vi "Trabalho.vi"() -> ()   [LabVIEW 2009]
uses:
  <vilib>/NXT/Block Support/NXT_InputPort.ctl
  <vilib>/NXT/Block Support/NXT_ButtonSelector.ctl
  <vilib>/NXT/Subs/MotorOutput.ctl
  <vilib>/NXT/Dual Mode Library/Waits/Wait_Num.vi
  <vilib>/NXT/Dual Mode Library/Display/drawText.vi
  <vilib>/NXT/Dual Mode Library/Sensors/Light_On.vi
  <vilib>/NXT/Dual Mode Library/Sensors/Sound_dB.vi
  <vilib>/NXT/Dual Mode Library/Sensors/Sonar_cm.vi
  <vilib>/NXT/Dual Mode Library/Sensors/readNXTButton.vi
  <vilib>/NXT/Dual Mode Library/Sensors/Touch_Pressed.vi
  <vilib>/NXT/Subs/NXT_SteeringOutputPort.ctl
panel:
  out "Verificacao":bool[](array[boolean])
  out "Cor Inicial":i16
  out "Toque\nPressionado":bool
  out "Visor":string
  out "Ruído":i16(slide) scale=0.0..100.0
  out "Luminosidade":i16
  out "Distância":i16
  out "Botao\nPressionado":bool
  # "O Mindstorms irá ficar no seguinte loop até que o botão central seja precionado:\nAciona os motores B e C para frente.\nMostrará os valores dos sensores na tela.\nCaso seja detectado: uma distância menor que 50cm, ou um ruído maior que 70dB, ou o sensor de toque seja precionado ou haja uma mudança de cor. O Mindstorms irá executar a seguinte rotina:\nIrá desligar os motores B e C.\nIrá ligar os motores B e C para trás e dará cinco voltas.\nSelecionará aleatoriamente um lado (direita/esquerda).\nEmitirá um som \"äleatório\".\nVirará 180 graus para o lado escolhido.\nE voltará ao loop."
  # "Configuração:\nOUT_A: GARRA\nOUT_B: RODA DA ESQUERDA\nOUT_C: RODA DA DIREITA\nIN_1: SENSOR DE TOQUE\nIN_2: SENSOR SONORO\nIN_3: SENSOR LUMINOSO\nIN_4: SENSOR ULTRA-SOM"
  # "1 - Distância menor que 50cm\n2 - Mudança de cor detectada\n3 - Ruído maior que 70dB\n4 - Toque precionado"
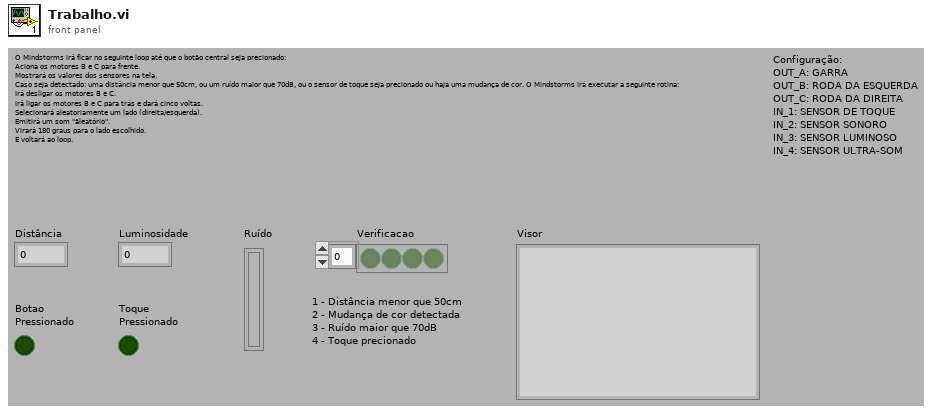
[diagram p1: front panel]
types:
  T1 = typedef "MotorOutput.ctl" = u8
  T2 = typedef "NXT_InputPort.ctl" = u8
  T3 = typedef "LVHSConnector.ctl" = cluster{"error":errorcluster, "address":string, "NXT #":i32, "Show Error":bool, "Connection":u16}
  T4 = typedef "NXT_SteeringOutputPort.ctl" = u16
  T5 = typedef "NXT_ButtonSelector.ctl" = u16
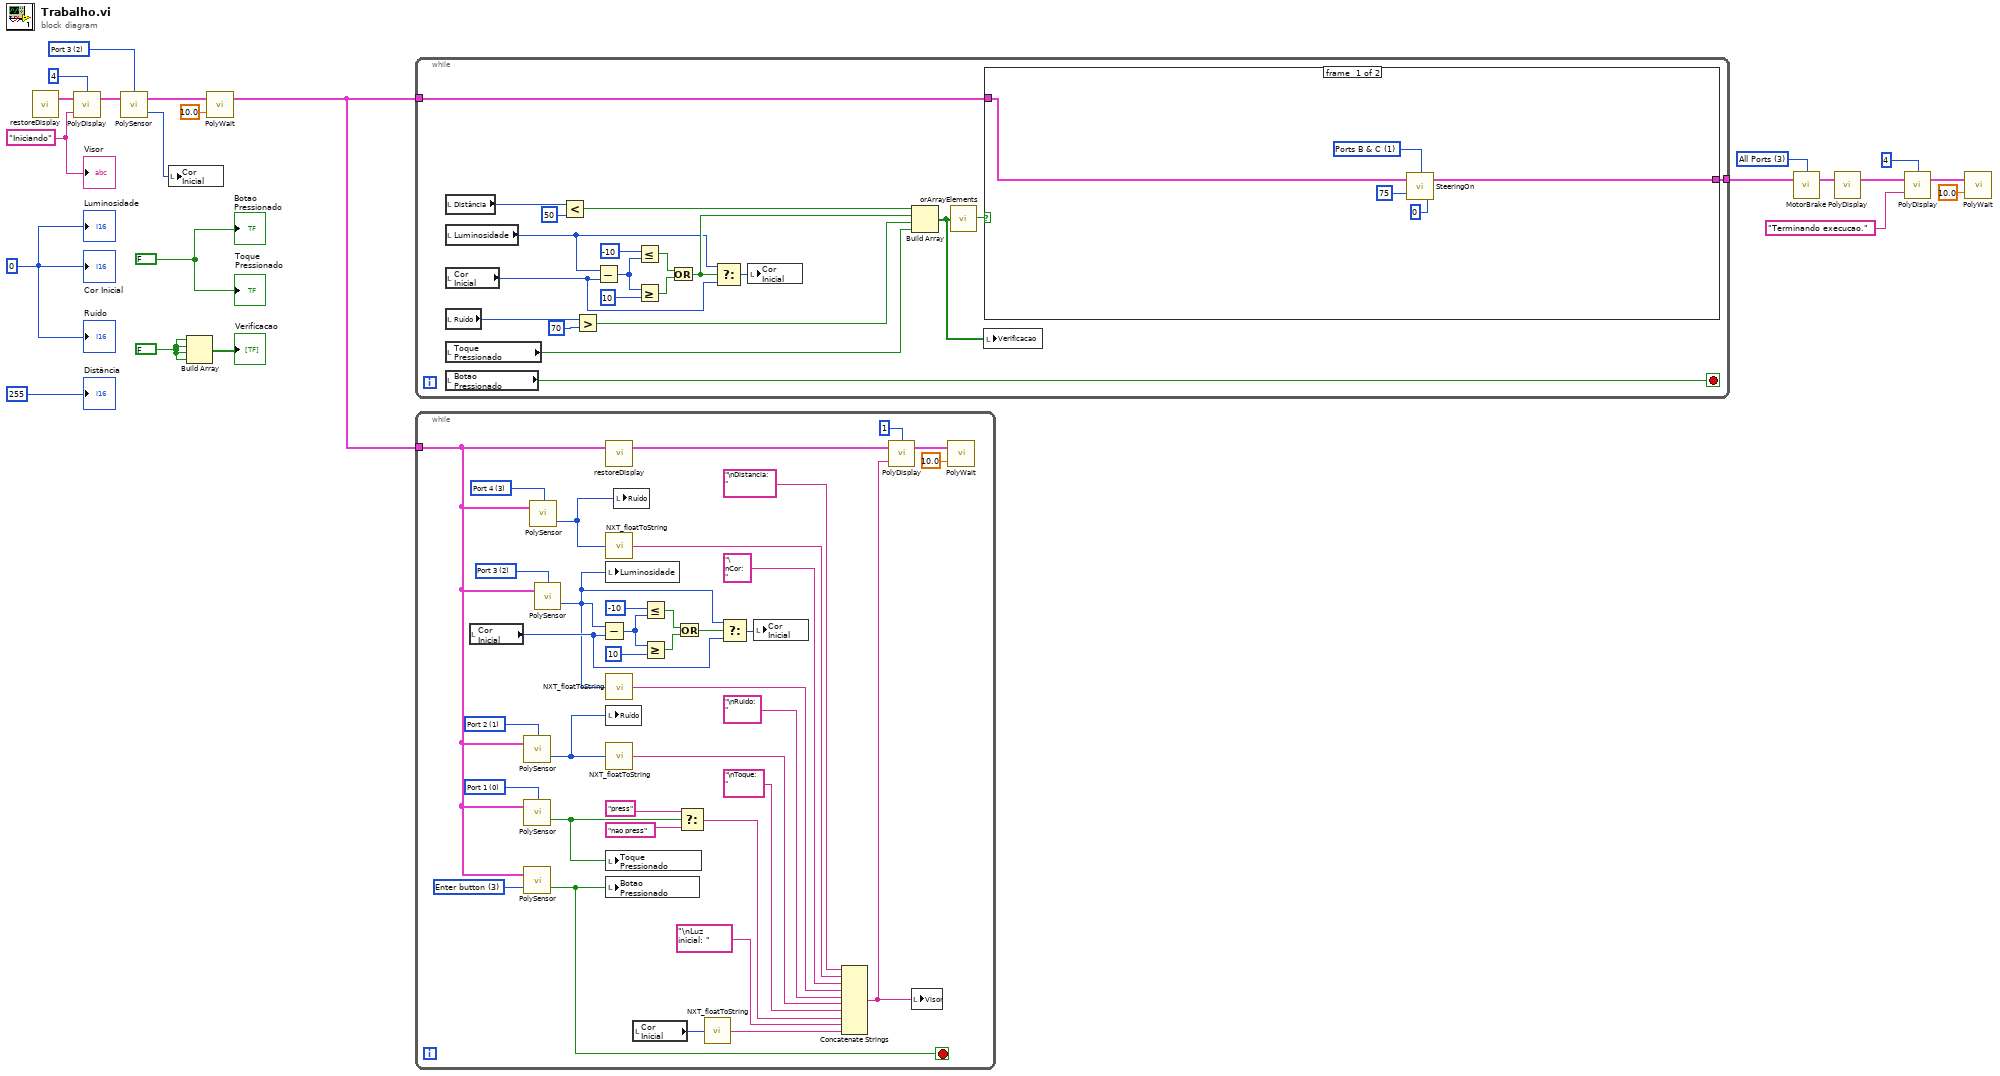
[diagram p0: block diagram]
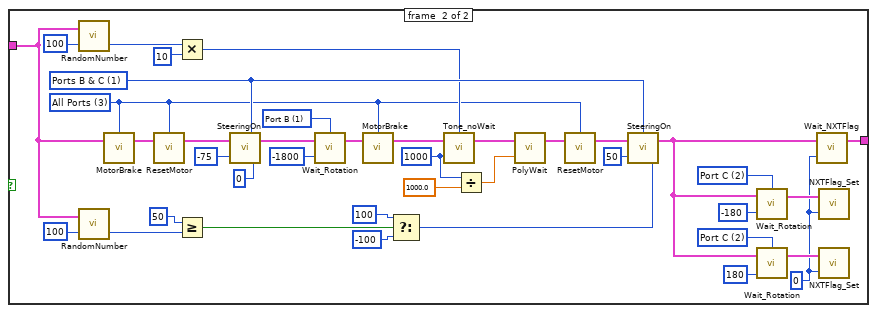
[diagram p2: hidden frame]
diagram:
  w2 = FALSE
  w14 = T1 3 items=["Port A", "Port B", "Port C", "All Ports"] ("Output Port (All Ports)")
  w10 = T2 2 items=["Port 1", "Port 2", "Port 3", "Port 4"] ("Input Port")
  w21 = "Iniciando"
  w20 = FALSE
  w5 = i16 0
  n1 = call <vilib>:"restoreDisplay.vi"() -> ("NXT"=w15:T3)  [unwired: 4 in]
  n2 = call-poly <vilib>:"PolyDisplay.vi"("Text"=w21, "NXT"=w15, "Line"=i16 4) -> ("NXT"=w6:T3)  [unwired: 1 in]
  n3 = call-poly <vilib>:"PolySensor.vi"("NXT"=w6, "Port (Port 3)"=w10) -> ("Scaled Value"=w9:i16, "NXT"=w7:T3)  [unwired: 1 in]
  n4 = local write "Cor Inicial"(w9) -> ()
  n5 = Build Array(w2, w2, w2, w2) -> (→"Verificacao":bool[])
  n6 = call-poly <vilib>:"PolyWait.vi"("Time (1 sec)"=sgl 10.0, "NXT"=w7) -> ("NXT"=w1:T3)  [unwired: 2 in]
  n7 = while {
    tunnel: w1 -> [w42]
    tunnel: [w41] -> w4
    stop <- w43 stop-if-true
    n8 = local read "Distância"() -> (w39:i16)
    n9 = local read "Luminosidade"() -> (w23:i16)
    n10 = local read "Cor Inicial"() -> (w30:i16)
    n11 = local read "Ruído"() -> (w27:i16)
    n12 = local read "Toque\nPressionado"() -> (w25:bool)
    n13 = local read "Botao\nPressionado"() -> (w43:bool)
    n14 = Less?(x=w39, y=i16 50) -> (x < y?=w37:bool)
    n15 = Greater?(x=w27, y=i16 70) -> (0:w26:bool)
    n16 = Subtract(x=w23, y=w30) -> (x-y=w34:i16)
    n17 = Less Or Equal?(x=i16 -10, y=w34) -> (x <= y?=w31:bool)
    n18 = Greater Or Equal?(x=w34, y=i16 10) -> (x >= y?=w32:bool)
    n19 = Or(x=w31, y=w32) -> (x .or. y?=w29:bool)
    n20 = Select(t=w23, s=w29, f=w30) -> (s? t:f=w36:i16)
    n21 = local write "Cor Inicial"(w36) -> ()
    n22 = Build Array(w37, w29, w26, w25) -> (w24:bool[])
    n23 = call <vilib>:"orArrayElements.vi"("Boolean Array"=w24) -> ("Logical OR"=w40:bool)
    n24 = local write "Verificacao"(w24) -> ()
    n25 = case shown="True" w40 {
      tunnel: w42 -> [w45 w84]
      tunnel: [w44 w49] -> w41
      frame #0 {
        w46 = T4 1 items=["Ports A & B", "Ports B & C", "Ports A & C"] ("Output Port")
        n26 = call <vilib>:"SteeringOn.vi"("Power (75)"=75, "Steering (100)"=0, "NXT"=w45, "Output Ports"=w46) -> ("NXT"=w44:T3)
      }
      frame #1 {
        w53 = u8 1 items=["Port A", "Port B", "Port C"] ("Output Port")
        w57 = i8 0
        w64 = T1 2 items=["Port A", "Port B", "Port C", "All Ports"] ("Output Port (All Ports)")
        w63 = T1 2 items=["Port A", "Port B", "Port C", "All Ports"] ("Output Port (All Ports)")
        w68 = u16 1000
        w50 = T1 3 items=["Port A", "Port B", "Port C", "All Ports"] ("Output Port (All Ports)")
        w83 = T4 1 items=["Ports A & B", "Ports B & C", "Ports A & C"] ("Output Port")
        n27 = call <vilib>:"RandomNumber.vi"("Max Value"=i16 100, "NXT"=w84) -> ("Random Number"=w79:u16)  [unwired: 1 in, 1 out]
        n28 = call <vilib>:"RandomNumber.vi"("Max Value"=i16 100, "NXT"=w84) -> ("Random Number"=w75:u16)  [unwired: 1 in, 1 out]
        n29 = call <vilib>:"MotorBrake.vi"("NXT"=w84, "Port (All Ports)"=w50) -> ("NXT"=w56:T3)  [unwired: 2 in]
        n30 = call <vilib>:"ResetMotor.vi"("NXT"=w56, "Port (All Ports)"=w50) -> ("NXT"=w55:T3)  [unwired: 2 in]
        n31 = Multiply(x=w79, y=u16 10) -> (x*y=w77:u16)
        n32 = Greater Or Equal?(x=u16 50, y=w75) -> (x >= y?=w74:bool)
        n33 = call <vilib>:"SteeringOn.vi"("Power (75)"=-75, "Steering (100)"=0, "NXT"=w55, "Output Ports"=w83) -> ("NXT"=w54:T3)
        n34 = call <vilib>:"Wait_Rotation.vi"("Position Change (180)"=-1800, "NXT"=w54, "Port (Port A)"=w53) -> ("NXT"=w65:T3)  [unwired: 1 in]
        n35 = call <vilib>:"MotorBrake.vi"("NXT"=w65, "Port (All Ports)"=w50) -> ("NXT"=w67:T3)  [unwired: 2 in]
        n36 = Select(t=100, s=w74, f=-100) -> (s? t:f=w76:i32)
        n37 = call <vilib>:"Tone_noWait.vi"("Duration (500 ms)"=w68, "NXT"=w67, "Tone (440 Hz)"=w77) -> ("NXT"=w81:T3)  [unwired: 1 in]
        n38 = Divide(x=w68, y=sgl 1000.0) -> (x/y=w70:sgl)
        n39 = call-poly <vilib>:"PolyWait.vi"("Time (1 sec)"=w70, "NXT"=w81) -> ("NXT"=w52:T3)  [unwired: 2 in]
        n40 = call <vilib>:"ResetMotor.vi"("NXT"=w52, "Port (All Ports)"=w50) -> ("NXT"=w51:T3)  [unwired: 2 in]
        n41 = call <vilib>:"SteeringOn.vi"("Power (75)"=50, "Steering (100)"=w76, "NXT"=w51, "Output Ports"=w83) -> ("NXT"=w58:T3)
        n42 = call <vilib>:"Wait_Rotation.vi"("Position Change (180)"=-180, "NXT"=w58, "Port (Port A)"=w63) -> ("NXT"=w59:T3)  [unwired: 1 in]
        n43 = call <vilib>:"Wait_Rotation.vi"("Position Change (180)"=180, "NXT"=w58, "Port (Port A)"=w64) -> ("NXT"=w60:T3)  [unwired: 1 in]
        n44 = call <vilib>:"Wait_NXTFlag.vi"("NXT Flag Number"=w57, "NXT"=w58) -> ("NXT"=w49:T3)  [unwired: 2 in]
        n45 = call <vilib>:"NXTFlag_Set.vi"("NXT Flag Number"=w57, "NXT"=w59) -> ()  [unwired: 2 in, 1 out]
        n46 = call <vilib>:"NXTFlag_Set.vi"("NXT Flag Number"=w57, "NXT"=w60) -> ()  [unwired: 2 in, 1 out]
      }
    }
  }
  n47 = while {
    tunnel: w1 -> [w89]
    stop <- w88 stop-if-true
    w106 = T5 3 items=["Enter button"=3, "Left button"=2, "Right button"=1] ("Button (Enter button)")
    w121 = T2 3 items=["Port 1", "Port 2", "Port 3", "Port 4"] ("Input Port")
    w122 = T2 2 items=["Port 1", "Port 2", "Port 3", "Port 4"] ("Input Port")
    w123 = T2 1 items=["Port 1", "Port 2", "Port 3", "Port 4"] ("Input Port")
    w124 = T2 0 items=["Port 1", "Port 2", "Port 3", "Port 4"] ("Input Port")
    n48 = local read "Cor Inicial"() -> (w94:i16)
    n49 = call-poly <vilib>:"PolySensor.vi"("NXT"=w89, "Port (Port 2)"=w123) -> ("Sound (dB)"=w91:i16)  [unwired: 1 in, 1 out]
    n50 = call-poly <vilib>:"PolySensor.vi"("NXT"=w89, "Port (Port 1)"=w124) -> ("Yes / No"=w90:bool)  [unwired: 1 in, 1 out]
    n51 = call-poly <vilib>:"PolySensor.vi"("Button (Enter button)"=w106, "NXT"=w89) -> ("Yes/No"=w88:bool)  [unwired: 1 in, 1 out]
    n52 = call-poly <vilib>:"PolySensor.vi"("NXT"=w89, "Port (Port 4)"=w121) -> ("Distance (cm)"=w101:i16)  [unwired: 1 in, 1 out]
    n53 = call-poly <vilib>:"PolySensor.vi"("NXT"=w89, "Port (Port 3)"=w122) -> ("Scaled Value"=w93:i16)  [unwired: 1 in, 1 out]
    n54 = Subtract(x=w93, y=w94) -> (x-y=w98:i16)
    n55 = call <vilib>:"restoreDisplay.vi"("NXT"=w89) -> ("NXT"=w105:T3)  [unwired: 3 in]
    n56 = call <vilib>:"NXT_floatToString.vi"("number"=w101) -> ("string"=w117:string)
    n57 = local write "Luminosidade"(w93) -> ()
    n58 = call <vilib>:"NXT_floatToString.vi"("number"=w93) -> ("string"=w115:string)
    n59 = local write "Ruído"(w91) -> ()
    n60 = call <vilib>:"NXT_floatToString.vi"("number"=w91) -> ("string"=w111:string)
    n61 = local write "Toque\nPressionado"(w90) -> ()
    n62 = local write "Botao\nPressionado"(w88) -> ()
    n63 = local write "Ruído"(w101) -> ()
    n64 = local read "Cor Inicial"() -> (w104:i16)
    n65 = Less Or Equal?(x=i16 -10, y=w98) -> (x <= y?=w95:bool)
    n66 = Greater Or Equal?(x=w98, y=i16 10) -> (x >= y?=w96:bool)
    n67 = Or(x=w95, y=w96) -> (x .or. y?=w92:bool)
    n68 = Select(t="press", s=w90, f="nao press") -> (s? t:f=w113:string)
    n69 = call <vilib>:"NXT_floatToString.vi"("number"=w104) -> ("string"=w102:string)
    n70 = Select(t=w93, s=w92, f=w94) -> (s? t:f=w100:i16)
    n71 = local write "Cor Inicial"(w100) -> ()
    n72 = Concatenate Strings("\nDistancia: ", w117, "\nCor: ", w115, "\nRuido: ", w111, "\nToque: ", w113, "\nLuz inicial: ", w102) -> (w107:string)
    n73 = call-poly <vilib>:"PolyDisplay.vi"("Text"=w107, "NXT"=w105, "Line"=i16 1) -> ("NXT"=w108:T3)  [unwired: 1 in]
    n74 = local write "Visor"(w107) -> ()
    n75 = call-poly <vilib>:"PolyWait.vi"("Time (1 sec)"=sgl 10.0, "NXT"=w108) -> ()  [unwired: 2 in, 1 out]
  }
  n76 = call <vilib>:"MotorBrake.vi"("NXT"=w4, "Port (All Ports)"=w14) -> ("NXT"=w12:T3)  [unwired: 2 in]
  n77 = call-poly <vilib>:"PolyDisplay.vi"("NXT"=w12) -> ("NXT"=w18:T3)  [unwired: 3 in]
  n78 = call-poly <vilib>:"PolyDisplay.vi"("Text"="Terminando execucao.", "NXT"=w18, "Line"=i16 4) -> ("NXT"=w11:T3)  [unwired: 1 in]
  n79 = call-poly <vilib>:"PolyWait.vi"("Time (1 sec)"=sgl 10.0, "NXT"=w11) -> ()  [unwired: 2 in, 1 out]
  "Botao\nPressionado" <- w20
  "Distância" <- i16 255
  "Luminosidade" <- w5
  "Ruído" <- w5
  "Visor" <- w21
  "Toque\nPressionado" <- w20
  "Cor Inicial" <- w5
